vi "Calculate joystick scaling.vi"(1 "Resolution factor X":i32=150, 2 "Resolution factor Y":i32=150, 3 "XPos max":i32=65535, 4 "YPos max":i32=65535, 6 "XPos min":i32, 7 "YPos min":i32) -> (8 "XPos Center":i32, 9 "YPos Center":i32, 10 "XPos Center scaled":i32, 11 "YPos Center scaled":i32, 12 "XPos min scaled":i32, 13 "YPos min scaled":i32, 14 "Scaling factor X":dbl format="%.2f", 15 "Scaling factor Y":dbl format="%.2f", 16 "XPos max scaled":i32, 17 "YPos max scaled":i32)   [LabVIEW 2026]
doc: "Sub-VI for operation with a joystick connected to the game port of the host computer. Calculates joystick position scaling. If Resolution factor * = *Pos max, maximum resolution is achieved. *Pos min and *Pos max depend on the Windows joystick calibration."
panel:
  # "Calculates joystick position scaling. If \"Resolution factor *\" = \"*Pos max\", \nmaximum resolution is achieved."
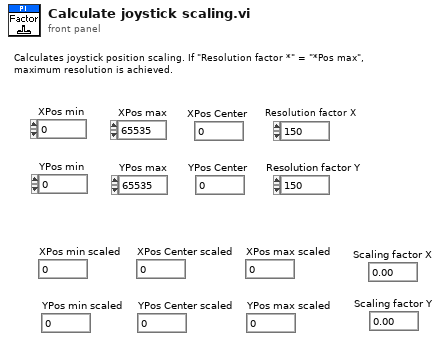
[diagram p1: front panel]
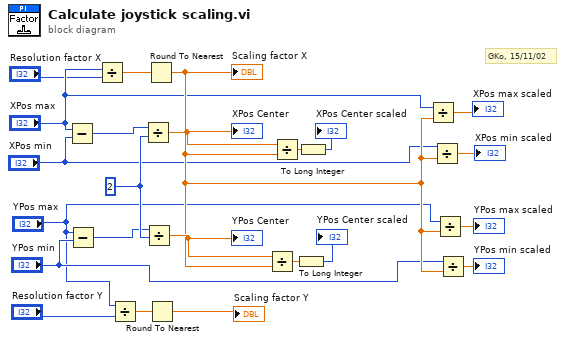
[diagram p0: block diagram]
diagram:
  w23 = 2 ("y")
  # "GKo, 15/11/02"
  n1 = Subtract(x="XPos max", y="XPos min") -> (x-y=w2:i32)
  n2 = Subtract(x="YPos max", y="YPos min") -> (x-y=w1:i32)
  n3 = Divide(x="XPos max", y="Resolution factor X") -> (x/y=w22:dbl)
  n4 = Divide(x="YPos max", y="Resolution factor Y") -> (x/y=w4:dbl)
  n5 = Divide(x=w2, y=w23) -> (x/y=w19:dbl)
  "XPos Center" <- w19
  n6 = Divide(x=w1, y=w23) -> (x/y=w18:dbl)
  "YPos Center" <- w18
  n7 = Round To Nearest(number=w22) -> (nearest integer value=w15:dbl)
  "Scaling factor X" <- w15
  n8 = Round To Nearest(number=w4) -> (nearest integer value=→"Scaling factor Y":dbl)
  n9 = Divide(x=w18, y=w15) -> (x/y=w20:dbl)
  n10 = Divide(x=w19, y=w15) -> (x/y=w21:dbl)
  n11 = To Long Integer(number=w20) -> (32bit integer=→"YPos Center scaled":i32)
  n12 = To Long Integer(number=w21) -> (32bit integer=→"XPos Center scaled":i32)
  n13 = Divide(x="XPos max", y=w15) -> (x/y=→"XPos max scaled":dbl)
  n14 = Divide(x="XPos min", y=w15) -> (x/y=→"XPos min scaled":dbl)
  n15 = Divide(x="YPos max", y=w15) -> (x/y=→"YPos max scaled":dbl)
  n16 = Divide(x="YPos min", y=w15) -> (x/y=→"YPos min scaled":dbl)
